vi "for_v0_v13.vi"() -> ()   [LabVIEW 2009]
panel:
  in  "d":dbl(knob)=4.861249431644813 scale=0.0..10.0
  out "Iteratia":dbl=26.0
  in  "stop":bool
  out "Picture":picture
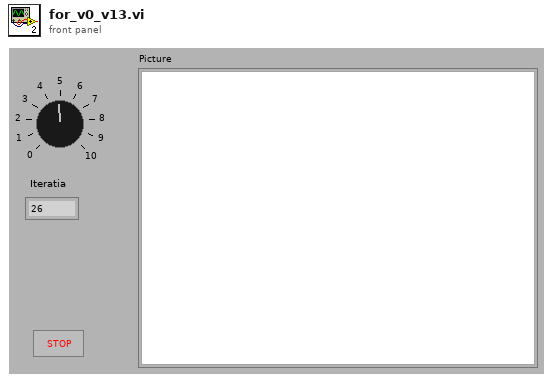
[diagram p1: front panel]
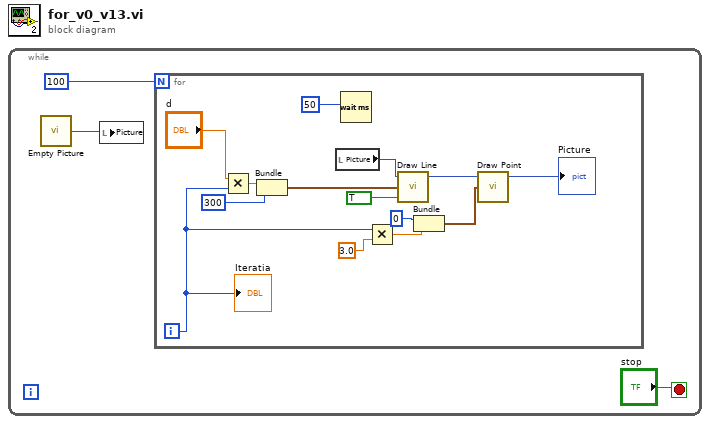
[diagram p0: block diagram]
diagram:
  n1 = while {
    stop <- "stop" stop-if-true
    n2 = call "Empty Picture"() -> ("empty picture"=w1:picture)
    n3 = local write "Picture"(w1) -> ()
    n4 = for {
      N: 100 -> [_]
      i -> [w5]
      n5 = Multiply(x="d", y=w5) -> (x*y=w9:dbl)
      n6 = Bundle(w9, 300) -> (w15:cluster{dbl, i32})  [unwired: 1 in]
      n7 = local read "Picture"() -> (w17:picture)
      n8 = Wait (ms)(milliseconds to wait=50) -> ()  [unwired: 1 out]
      n9 = Multiply(x=w5, y=3.0) -> (x*y=w6:dbl)
      n10 = call <vilib>:"Draw Line.vi"("picture"=w17, "end point"=w15, "absolute coordinates?(T)"=TRUE) -> ("new picture"=w16:picture)  [unwired: 6 in]
      n11 = Bundle(0, w6) -> (w8:cluster{i32, dbl})  [unwired: 1 in]
      n12 = call <vilib>:"Draw Point.vi"("picture"=w16, "point(x,y)"=w8) -> ("new picture"=→"Picture":picture)  [unwired: 7 in]
      "Iteratia" <- w5
    }
  }
